vi "Orb_DeRegister.vi"(0 "error in (no error)":errorcluster, 6 "De-registering VI":string) -> (3 "error out":errorcluster)   [LabVIEW 2009]
uses:
  Orb_Global.vi
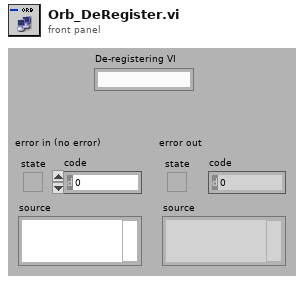
[diagram p1: front panel]
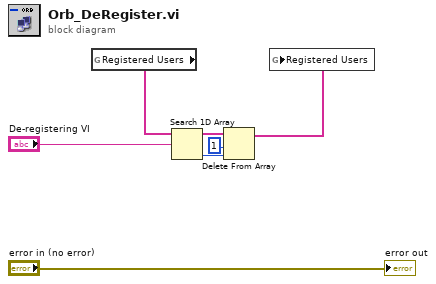
[diagram p0: block diagram]
diagram:
  n1 = global read "Orb_Global.vi" "Registered Users"() -> (w5:string[])
  n2 = Search 1D Array(1D array=w5, element="De-registering VI") -> (index of element=w4:i32)  [unwired: 1 out]
  n3 = Delete From Array(array=w5, length=1 ("longueur"), index=w4) -> (array with subset deleted=w2:string[])  [unwired: 1 out]
  n4 = global write "Orb_Global.vi" "Registered Users"(w2) -> ()
  "error out" <- "error in (no error)"
